vi "RG DAQ control for PIA.vi"(7 "LED line":tag, 8 "error in":errorcluster, 11 "value":bool) -> (0 "error out":errorcluster)   [LabVIEW 2017]
uses:
  <vilib>/DAQmx/write.llb/DAQmx Write.vi
  <vilib>/DAQmx/write.llb/DAQmx Write (Digital 1D Bool NChan 1Samp 1Line).vi
  <vilib>/DAQmx/create/channels.llb/DAQmx Create Channel (DO-Digital Output).vi
  <vilib>/DAQmx/miscellaneous.llb/DAQmx Fill In Error Info.vi
  <resource>/objmgr/daqmx.rc
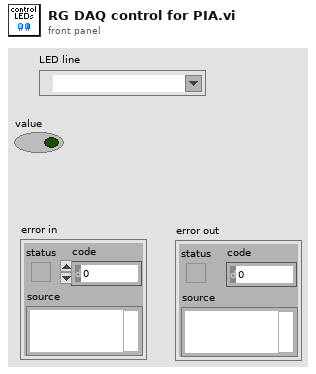
[diagram p1: front panel]
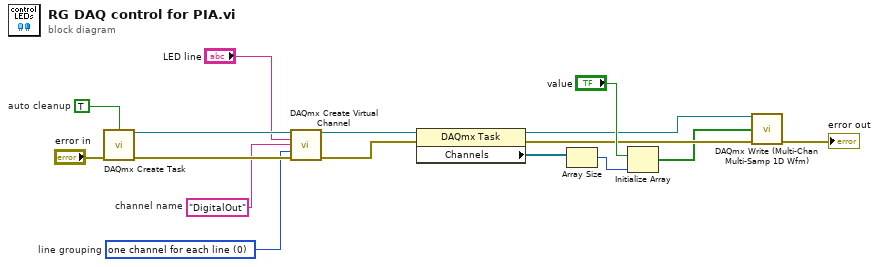
[diagram p0: block diagram]
diagram:
  w12 = 0 items=["one channel for each line", "one channel for all lines"]  # line grouping
  w11 = "DigitalOut"  # channel name
  w14 = TRUE  # auto cleanup
  n1 = call <vilib>:"DAQmx Create Task.vi"("auto cleanup"=w14, "error in"="error in") -> ("task out"=w13:refnum<k21>, "error out"=w15:errorcluster)  [unwired: 12 in]
  n2 = call-poly <vilib>:"DAQmx Create Virtual Channel.vi"("task in"=w13, "lines"="LED line", "name to assign"=w11, "line grouping"=w12, "error in"=w15) -> ("task out"=w8:refnum<k21>, "error out"=w7:errorcluster)  [unwired: 9 in]
  n3 = property class="DAQmx Task"(reference=w8, error in=w7) -> (reference out=w5:refnum<k21>, error out=w4:errorcluster, "Channels"=w10:refnum<k21>[])
  n4 = Array Size(array=w10) -> (size(s)=w9:i32)
  n5 = Initialize Array("value", w9) -> (w3:bool[])
  n6 = call-poly "DAQmx Write (Multi-Chan Multi-Samp 1D Wfm).vi"("task/channels in"=w5, "data"=w3, "error in"=w4) -> ("error out"=→"error out":errorcluster)  [unwired: 10 in, 2 out]
